vi "DSF.Shared.Configuration.Plugin.Validate.vi"(8 "error in (no error)":errorcluster, 11 "Plugin Configuration in":refnum<class "DSF.Shared.Configuration.Plugin.lvclass">) -> (0 "error out":errorcluster, 3 "Plugin Configuration out":refnum<class "DSF.Shared.Configuration.Plugin.lvclass">)   [LabVIEW 2017, in "DSF.Shared.lvlib" / "DSF.Shared.Configuration.Plugin.lvclass"]
uses:
  DSF.Shared.Configuration.Plugin.lvclass
  DSF.Shared.Configuration.Plugin.lvclass/DSF.Shared.Configuration.Plugin.ctl
  Transfer Group/DSF.Shared.Configuration.Transfer Group.lvclass
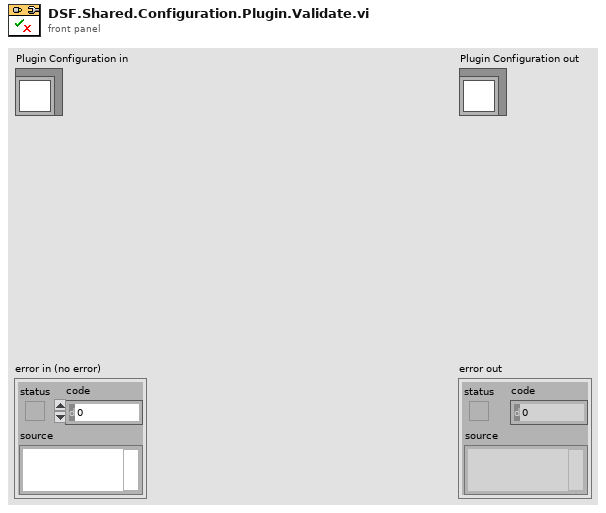
[diagram p1: front panel]
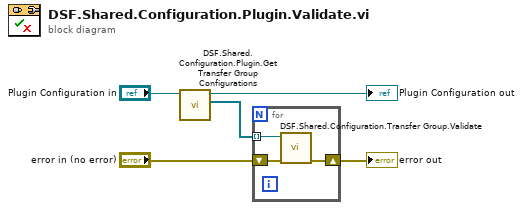
[diagram p0: block diagram]
diagram:
  n1 = call "DSF.Shared.Configuration.Plugin.Get Transfer Group Configurations.vi"("Plugin Configuration in"="Plugin Configuration in") -> ("Transfer Group Configurations"=w4:refnum<class "DSF.Shared.Configuration.Transfer Group.lvclass">[], "Plugin Configuration out"=→"Plugin Configuration out":refnum<class "DSF.Shared.Configuration.Plugin.lvclass">)  [unwired: 9 in]
  n2 = for {
    tunnel: w4 -> [w8] mode=indexing
    shift-right: [w6] -> w2
    shift-left: "error in (no error)" -> [w7]
    n3 = call "DSF.Shared.Configuration.Transfer Group.Validate.vi"("error in (no error)"=w7, "Transfer Group Configuration in"=w8) -> ("error out"=w6:errorcluster)  [unwired: 8 in, 1 out]
  }
  "error out" <- w2
